vi "Decompose VI (Path).vi"(8 "error in (no error)":errorcluster, 11 "VI path":path) -> (0 "error out":errorcluster, 1 "Block Diagram XML":string, 2 "Front Panel XML":string, 3 "VI path out":path, 4 "Other resources":T1[](array[typedef]))   [LabVIEW 2026, in "VILab.lvlib"]
uses:
  VILab.lvlib
  CTLs/Resource.ctl
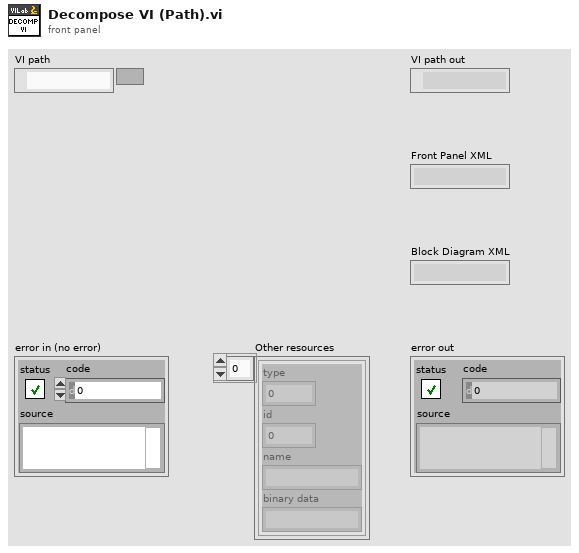
[diagram p1: front panel]
types:
  T1 = typedef "VILab.lvlib/Resource.ctl" = cluster{"type":u32, "id":i32, "name":string, "binary data":string}
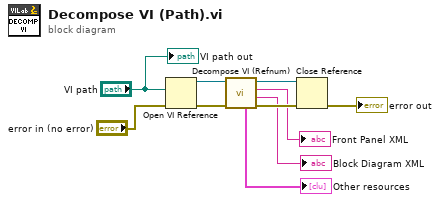
[diagram p0: block diagram]
diagram:
  n1 = Open VI Reference(vi path="VI path", error in (no error)="error in (no error)") -> (vi reference=w10:refnum<vi>, error out=w9:errorcluster)  [unwired: 4 in]
  n2 = call "Decompose VI (Refnum).vi"("error in (no error)"=w9, "VI Ref"=w10) -> ("error out"=w6:errorcluster, "Block Diagram XML"=→"Block Diagram XML":string, "Front Panel XML"=→"Front Panel XML":string, "VI Ref out"=w7:refnum<vi>, "Other resources"=→"Other resources":T1[])  [unwired: 5 in]
  n3 = Close Reference(reference=w7, error in (no error)=w6) -> (error out=→"error out":errorcluster)
  "VI path out" <- "VI path"
